vi "LuaVIEW Compile.vi"(0 "script name":string, 5 "LuaVIEW reference in":T1, 7 "script":string, 11 "error in (no error)":errorcluster) -> (6 "LuaVIEW reference out":T1, 15 "error out":errorcluster)   [LabVIEW 2013]
doc: "Compiles the provided script string so that it can be executed. This is not compilation to native machine code but rather compilation to bytecode that can execute on the Lua virtual machine instance associated with the provided LuaVIEW reference. Multiple scripts can be compiled. These will be executed in order of compilation."
uses:
  typedefs/t_LuaVIEW Reference.ctl
  typedefs/et_LuaVIEW CIN Actions.ctl
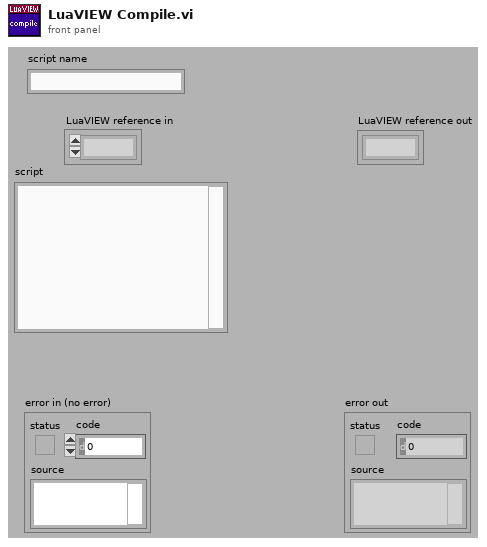
[diagram p1: front panel]
types:
  T1 = typedef "t_LuaVIEW Reference.ctl" = refnum<k1>
  T2 = typedef "et_LuaVIEW CIN Actions.ctl" = enum16{"checksynopsis", "_open", "_registerpublic", "_registerexport", "__never_an_error_result_ns", "luaversion", "cinversion", "_totals", "_taskcount", "pathological", "_unregnextpublic", "registryusecount", "__per_state_actions", "regsetprivate", "regsetindex", "regsetmodule", "_revokeexports", "_usepublic", "prepare", "compile", "execute", "call", "unregstaterefs", "_close", "pullboolean", "pullnumber", "pullI8", "pullU8", "pullI16", "pullU16", "pullI32", "pullU32", "pullobject", "pullrefnum", "pullstring", "pullflat", "pushflat", "pushobject", "getattribute", "setattribute", "stacktostring", "_startyieldtest", "_endyieldtest", "_pollprintbuffer", "__never_an_error_result_ps", "_pollexport", "setclone", "forcecleanup", "gettop", "clearstack", "insert", "pushboolean", "pushnumber", "pushrefnum", "pushstring", "pushnil", "pushvalue", "gettaskref", "settaskref"}
  T3 = typedef "et_LuaVIEW CIN Results.ctl" = enum16{"OK", "error", "main", "call", "clonecall", "modulecall", "exportcall", "index", "yield"}
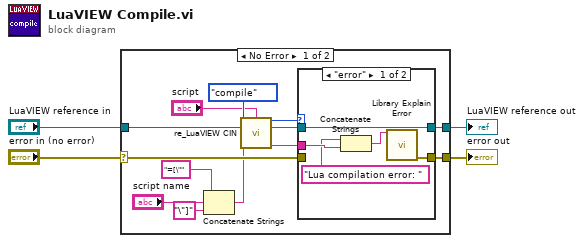
[diagram p0: block diagram]
diagram:
  n1 = case shown="No Error" "error in (no error)" {
    selector: "error in (no error)" -> [w11 w26]
    tunnel: [w10 w25] -> w4
    tunnel: [w17 w26] -> w3
    tunnel: "LuaVIEW reference in" -> [w16 w25]
    frame No Error {
      n2 = Concatenate Strings("=[\"", "script name", "\"]") -> (w7:string)
      n3 = call "re_LuaVIEW CIN.vi"("action"=et_LuaVIEW_CIN_Actions."compile", "supplement"="script", "LuaVIEW reference in"=w16, "string in"=w7) -> ("result"=w14:T3, "LuaVIEW reference out"=w12:T1, "string out"=w13:string)  [unwired: 5 in, 4 out]
      n4 = case shown="\"error\"" w14 {
        tunnel: w13 -> [w19 _]
        tunnel: [w22 w23] -> w17
        tunnel: w12 -> [w21 w24]
        tunnel: [w21 w24] -> w10
        tunnel: w11 -> [_ w23]
        frame "error" {
          n5 = Concatenate Strings("Lua compilation error: " ("string"), w19) -> (w20:string)
          n6 = call "Library Explain Error.vi"("explanation prefix (none)"=w20) -> ("explained error"=w22:errorcluster)  [unwired: 14 in]
        }
        frame Default {
        }
      }
    }
    frame Error {
    }
  }
  "LuaVIEW reference out" <- w4
  "error out" <- w3
